vi "(x,y) to XY.vi"   [LabVIEW 2019, in "xy_utilities.lvlib"]
doc: "Convert <b>(x,y)</b> coordinates (array of clusters of (x,y) values) to <b>XY-data</b> (cluster of arrays of X and Y).\n\nWire data to the data input to determine the polymorphic instance to use or manually select the instance."
uses:
  xy_utilities.lvlib
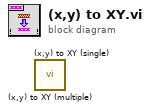
[diagram p0: block diagram]
diagram:
  n1 = call "(x,y) to XY (multiple).vi"() -> ()  [unwired: 10 in, 2 out]
  n2 = call "(x,y) to XY (single).vi"() -> ()  [unwired: 10 in, 2 out]
